vi "GetCurrent.vi"(4 "error in":errorcluster, 5 "connection ID":refnum<k5>) -> (0 "Current":string, 1 "error out":errorcluster, 2 "connection ID out":refnum<k5>, 3 "Answer":bool)   [LabVIEW 2013]
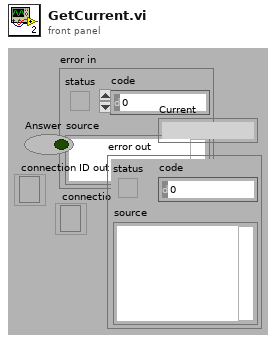
[diagram p1: front panel]
types:
  T1 = enum16{"Standard", "Buffered", "CRLF", "Immediate"}
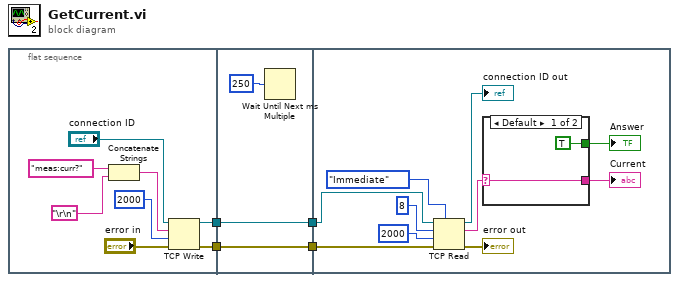
[diagram p0: block diagram]
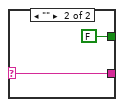
[diagram p2: hidden frame]
diagram:
  n1 = flat-sequence {
    tunnel: [w9] -> w3
    tunnel: [w8] -> w1
    tunnel: [w14] -> w4
    tunnel: w3 -> [w14]
    tunnel: [w13] -> w2
    tunnel: w1 -> [w13]
    tunnel: w4 -> [w17]
    tunnel: w2 -> [w16]
    frame #0 {
      n2 = Concatenate Strings("meas:curr?" ("data in"), "\r\n") -> (w6:string)
      n3 = TCP Write(connection ID="connection ID", data in=w6, error in (no error)="error in", 9:2000 ("timeout ms (25000)")) -> (connection ID out=w9:refnum<k5>, error out=w8:errorcluster)  [unwired: 1 out]
    }
    frame #1 {
      n4 = Wait Until Next ms Multiple(millisecond multiple=u32 250) -> ()  [unwired: 1 out]
    }
    frame #2 {
      n5 = TCP Read(connection ID=w17, bytes to read=8, error in (no error)=w16, 7:T1."Immediate" ("mode (standard)"), 9:2000 ("timeout ms (25000)")) -> (connection ID out=→"connection ID out":refnum<k5>, data out=w23:string, error out=→"error out":errorcluster)
      n6 = case shown="Default" w23 {
        selector: w23 -> [w27 w29]
        tunnel: [w27 w29] -> w22
        tunnel: [TRUE FALSE] -> w21
        frame Default {
        }
        frame "" {
        }
      }
      "Current" <- w22
      "Answer" <- w21
    }
  }
